vi "Scale Acquired Data PXIe.vi"(6 "range (V)":ext=2.0, 9 "Sample Rate":dbl=100000000.0, 10 "Number of Bits":i16=14, 11 "Data In":ext[](array[numeric])) -> (2 "EXT_Values":ext[](array[numeric]), 3 "Data Out":waveform(dbl)={"t0"=timestamp(0 s since 1904-01-01), "dt"=1e-08, "Y"=[]})   [LabVIEW 2018]
doc: "This VI scales the raw data returned by the adapter module from ADC codes to volts. It also stores the data in a waveform data type and sets the sample rate for the waveform."
panel:
  # "Refer to the Block Diagram of this VI for execution comments."
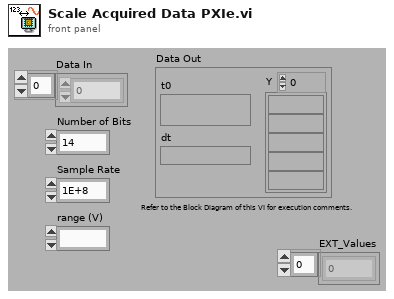
[diagram p1: front panel]
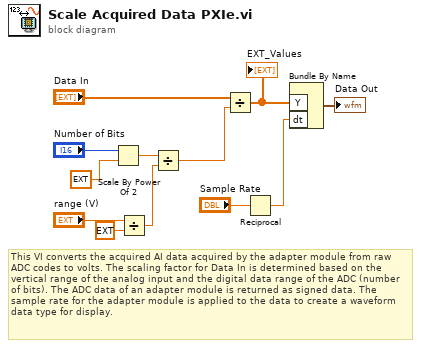
[diagram p0: block diagram]
diagram:
  # "This VI converts the acquired AI data acquired by the adapter module from raw ADC codes to volts. The scaling factor for Data In is determined based on the vertical range of the analog input and the digital data range of the ADC (number of bits). The ADC data of an adapter module is returned as signed data. The sample rate for the adapter module is applied to the data to create a waveform data type for display."
  n1 = Scale By Power Of 2(n="Number of Bits", x=ext 0.5) -> (x*2^n=w1:ext)
  n2 = Divide(x="range (V)", y=ext 2.0) -> (x/y=w2:ext)
  n3 = Divide(x=w1, y=w2) -> (x/y=w6:ext)
  n4 = Divide(x="Data In", y=w6) -> (x/y=w10:ext[])
  "EXT_Values" <- w10
  n5 = Reciprocal(x="Sample Rate") -> (1/x=w9:dbl)
  n6 = Bundle By Name("Y"=w10, "dt"=w9) -> (→"Data Out":waveform(ext))  [unwired: 1 out]
